vi "Get Process Handle.vi"(8 "error in (no error)":errorcluster, 10 "processName":string="SeqEdit", 11 ".NET Refnum in":refnum<k24>) -> (0 "error out":errorcluster, 2 "target process handle":refnum<k24>, 3 ".NET Refnum out":refnum<k24>)   [LabVIEW 2016]
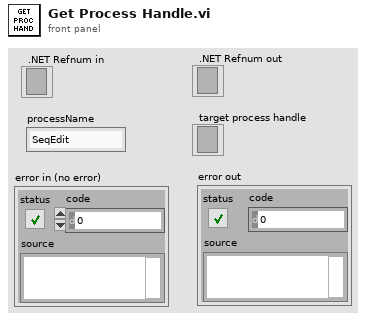
[diagram p1: front panel]
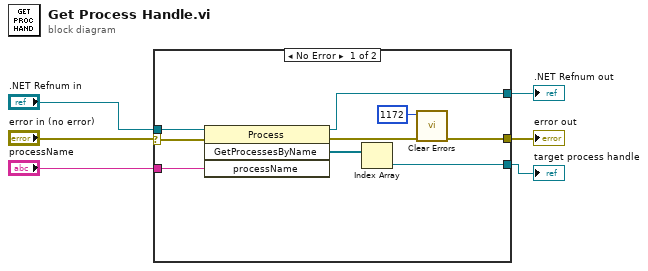
[diagram p0: block diagram]
diagram:
  n1 = case shown="No Error" "error in (no error)" {
    selector: "error in (no error)" -> [w9 w16]
    tunnel: [w15 _] -> w6
    tunnel: [w8 w16] -> w5
    tunnel: [w13 _] -> w4
    tunnel: "processName" -> [w11 _]
    tunnel: ".NET Refnum in" -> [w10 _]
    frame No Error {
      n2 = invoke class="Process" method="GetProcessesByName"(reference=w10, error in=w9, "processName"=w11) -> (reference out=w13:refnum<k24>, error out=w14:errorcluster, "GetProcessesByName"=w12:refnum<k24>[])  [unwired: 1 in, 1 out]
      n3 = Index Array(array=w12) -> (element=w15:refnum<k24>)  [unwired: 1 in]
      n4 = call <vilib>:"Clear Errors.vi"("error in (no error)"=w14, "specific error code to clear (0: all)"=1172) -> ("error out"=w8:errorcluster)  [unwired: 4 in, 1 out]
    }
    frame Error {
    }
  }
  ".NET Refnum out" <- w4
  "error out" <- w5
  "target process handle" <- w6
